vi "EncodeTermination.vi"(11 "String in":string) -> (3 "String out":string)   [LabVIEW 2015, in "Nav6.lvlib"]
uses:
  Nav6.lvlib
panel:
  out "length":i32
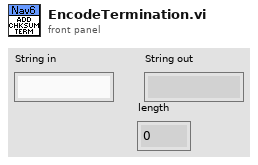
[diagram p1: front panel]
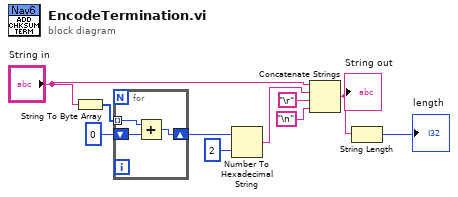
[diagram p0: block diagram]
diagram:
  n1 = String To Byte Array(string="String in") -> (unsigned byte array=w8:u8[])
  n2 = for {
    tunnel: w8 -> [w12] mode=indexing
    shift-right: [w11] -> w6
    shift-left: u8 0 -> [w13]
    n3 = Add(x=w12, y=w13) -> (x+y=w11:u8)
  }
  n4 = Number To Hexadecimal String(1:i16 2 ("width (-)"), 2:w6) -> (0:w5:string)
  n5 = Concatenate Strings("String in", w5, "\r", "\n") -> (w4:string)
  "String out" <- w4
  n6 = String Length(string=w4) -> (length=→"length":i32)
